vi "AddBus.vi"(6 "ShowPanel? (f)":bool=TRUE, 7 "BusNumber":i32, 8 "ErrorIn":errorcluster[](array[cluster]), 10 "ModuleList":string[](array[string]), 11 "Bus.lvclass":refnum<class "Bus.lvclass">) -> (0 "ErrorOut":errorcluster[](array[cluster]), 2 "UsrEvents":variant[](array[variant]), 3 "Bus.lvclass":refnum<class "Bus.lvclass">)   [LabVIEW 2018, in "Bus.lvclass"]
uses:
  Bus.lvclass
  Bus.lvclass/Bus.ctl
  TestClass/Test.lvclass/Test.ctl
  TestClass/Test.lvclass
  TestClass/Accessors/Read ErrorSeverity.vi
  Accessors/Write BusNumber.vi
  Accessors/Write Test.vi
  Accessors/Read BusNumber.vi
  Accessors/Read Test.vi
  <vilib>/Utility/error.llb/Error Cluster From Error Code.vi
  <vilib>/ErrorRing/Error Ring.xnode
  <userlib>/NIST/NISTErrorLib/NISTErrorLib.lvlib
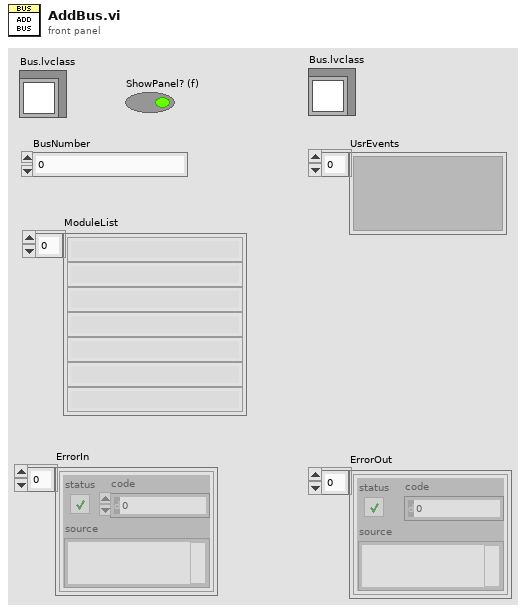
[diagram p1: front panel]
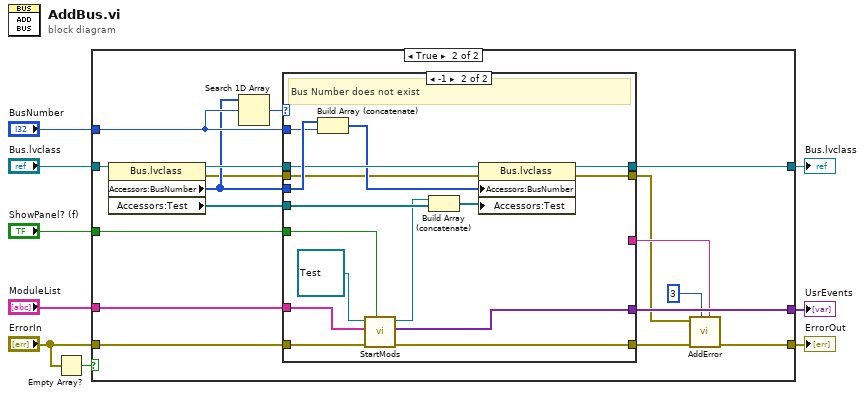
[diagram p0: block diagram]
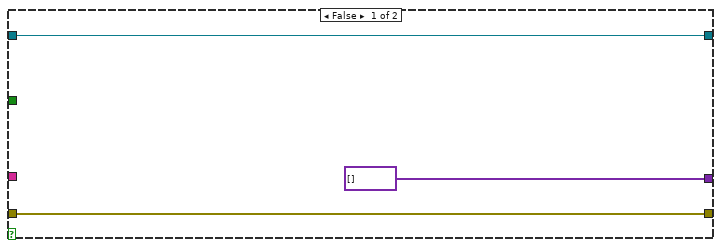
[diagram p2: hidden frame]
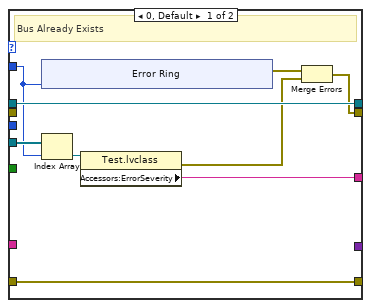
[diagram p3: hidden frame]
diagram:
  n1 = Empty Array?(array="ErrorIn") -> (empty?=w8:bool)
  n2 = case shown="True" w8 {
    tunnel: "ErrorIn" -> [w12 w24]
    tunnel: [w12 w15] -> w7
    tunnel: "Bus.lvclass" -> [w11 w29]
    tunnel: [w11 w23] -> w5
    tunnel: "BusNumber" -> [_ w22]
    tunnel: "ModuleList" -> [_ w28]
    tunnel: [variant[] [] ("Events") w26] -> w2
    tunnel: "ShowPanel? (f)" -> [_ w19]
    frame False {
    }
    frame True {
      n3 = property class="Bus.lvclass"(reference=w29) -> (reference out=w25:refnum<class "Bus.lvclass">, error out=w18:errorcluster, "Accessors:BusNumber"=w21:i32[], "Accessors:Test"=w27:refnum<class "Test.lvclass">[])  [unwired: 1 in]
      n4 = Search 1D Array(1D array=w21, element=w22) -> (index of element=w20:i32)  [unwired: 1 in]
      n5 = case shown="-1" w20 {
        tunnel: w21 -> [_ w61]
        tunnel: w22 -> [w36 w60]
        tunnel: w28 -> [_ w58]
        tunnel: w27 -> [w37 w57]
        tunnel: [_ w55] -> w26
        tunnel: w25 -> [w38 w54]
        tunnel: w24 -> [w34 w51]
        tunnel: [w34 w50] -> w16
        tunnel: [w38 w49] -> w23
        tunnel: w19 -> [_ w48]
        tunnel: w18 -> [_ w47]
        tunnel: [w30 w46] -> w13
        tunnel: [w33 _] -> w14
        frame 0, Default {
          # "Bus Already Exists"
          n6 = xnode "Error Ring"("parameter 0"=w36) -> ("error out"=w32:errorcluster)
          n7 = Index Array(array=w37, index=w36) -> (element=w35:refnum<class "Test.lvclass">)
          n8 = property class="Test.lvclass"(reference=w35) -> (error out=w31:errorcluster, "Accessors:ErrorSeverity"=w33:string)  [unwired: 1 in, 1 out]
          n9 = Merge Errors(w32, w31) -> (w30:errorcluster)
        }
        frame -1 {
          # "Bus Number does not exist"
          n10 = Build Array (concatenate)(w61, w60) -> (w53:i32[])
          n11 = call "StartMods.vi"("ShowPanel? (f)"=w48, "ErrorArray"=w51, "ModuleList"=w58, "Test.lvclass"=refnum<class "Test.lvclass"> refnum) -> ("ErrorArray"=w50:errorcluster[], "Events"=w55:variant[], "Test.lvclass"=w56:refnum<class "Test.lvclass">)  [unwired: 5 in]
          n12 = Build Array (concatenate)(w56, w57) -> (w52:refnum<class "Test.lvclass">[])
          n13 = property class="Bus.lvclass"(reference=w54, error in=w47, "Accessors:BusNumber"=w53, "Accessors:Test"=w52) -> (reference out=w49:refnum<class "Bus.lvclass">, error out=w46:errorcluster)
        }
      }
      n14 = call <userlib>:"AddError.vi"("Severity"=w14, "Priority"=u8 3, "ErrorArray"=w16, "error in (no error)"=w13) -> ("ErrorArray"=w15:errorcluster[])  [unwired: 6 in, 1 out]
    }
  }
  "Bus.lvclass" <- w5
  "ErrorOut" <- w7
  "UsrEvents" <- w2
